vi "Convert Byte Range to Range Header.vi"(11 "Range":T2) -> (3 "Range Header":T1={"name"="User-Agent", "value"=""})   [LabVIEW 2015, in "NI_AWS_Core.lvlib"]
uses:
  NI_AWS_Core.lvlib
  Request Range.ctl
  HTTP Request/Name Value Pair.ctl
  HTTP Request/HTTP Request.lvclass
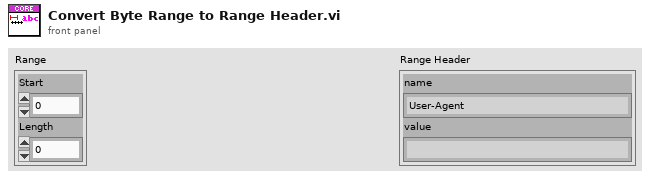
[diagram p1: front panel]
types:
  T1 = typedef "NI_AWS_Core.lvlib/HTTP Request.lvclass/Name Value Pair.ctl" = cluster{"name":string, "value":string}
  T2 = typedef "NI_AWS_Core.lvlib/Request Range.ctl" = cluster{"Start":i64, "Length":i64}
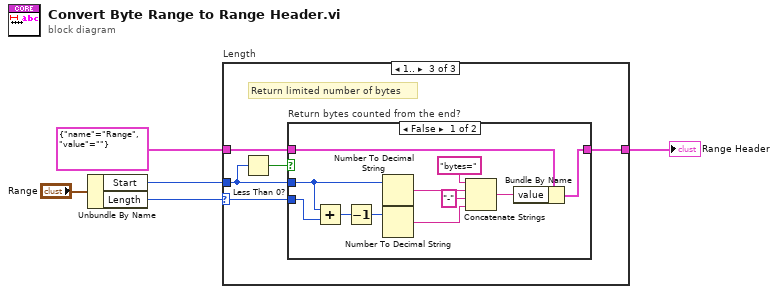
[diagram p0: block diagram]
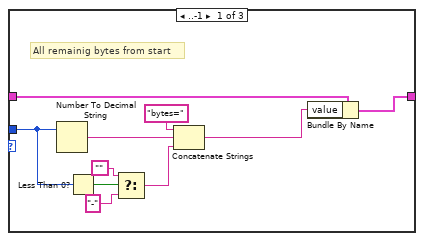
[diagram p2: hidden frame]
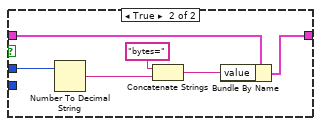
[diagram p4: hidden frame]
diagram:
  n1 = Unbundle By Name("Range") -> ("Start"=w3:i64, "Length"=w4:i64)
  n2 = case "Length" shown="1.." w4 {
    selector: w4 -> [_ _ w20]
    tunnel: w3 -> [w10 _ w19]
    tunnel: T1 {"name"="Range", "value"=""} ("Name Value Pair") -> [w15 w16 w18]
    tunnel: [w14 w16 w17] -> w1
    frame ..-1 {
      # "All remainig bytes from start"
      n3 = Number To Decimal String(number=w10) -> (decimal integer string=w13:string)  [unwired: 1 in]
      n4 = Less Than 0?(x=w10) -> (x < 0?=w9:bool)
      n5 = Select(t="", s=w9, f="-" ("string")) -> (s? t:f=w6:string)
      n6 = Concatenate Strings("bytes=" ("string"), w13, w6) -> (w11:string)
      n7 = Bundle By Name(cluster=w15, "value"=w11) -> (w14:T1)
    }
    frame 0 {
      # "Return nothing???!!! -> return everything!"
    }
    frame 1.. {
      # "Return limited number of bytes"
      n8 = Less Than 0?(x=w19) -> (x < 0?=w21:bool)
      n9 = case "Return bytes counted from the end?" shown="False" w21 {
        tunnel: w20 -> [w32 _]
        tunnel: w19 -> [w31 w38]
        tunnel: w18 -> [w26 w37]
        tunnel: [w24 w33] -> w17
        frame False {
          n10 = Add(x=w31, y=w32) -> (x+y=w23:i64)
          n11 = Decrement(x=w23) -> (x-1=w22:i64)
          n12 = Number To Decimal String(number=w31) -> (decimal integer string=w30:string)  [unwired: 1 in]
          n13 = Number To Decimal String(number=w22) -> (decimal integer string=w27:string)  [unwired: 1 in]
          n14 = Concatenate Strings("bytes=" ("string"), w30, "-" ("string"), w27) -> (w25:string)
          n15 = Bundle By Name(cluster=w26, "value"=w25) -> (w24:T1)
        }
        frame True {
          n16 = Number To Decimal String(number=w38) -> (decimal integer string=w36:string)  [unwired: 1 in]
          n17 = Concatenate Strings("bytes=" ("string"), w36) -> (w34:string)
          n18 = Bundle By Name(cluster=w37, "value"=w34) -> (w33:T1)
        }
      }
    }
  }
  "Range Header" <- w1
